vi "Get Actor Core Control Labels.vi"(8 "error in":errorcluster, 11 "Class in":refnum<class>) -> (0 "error out":errorcluster, 2 "Labels":string[](array[string]), 3 "Class out":refnum<class>)   [LabVIEW 2023, in "Label-Driven UI.lvlib"]
doc: "Actor Core.vi에 포함되어 있는 Nested in 컨트롤과 error in 컨트롤을 제외한 모든 컨트롤의 라벨들을 얻습니다."
uses:
  Label-Driven UI.lvlib
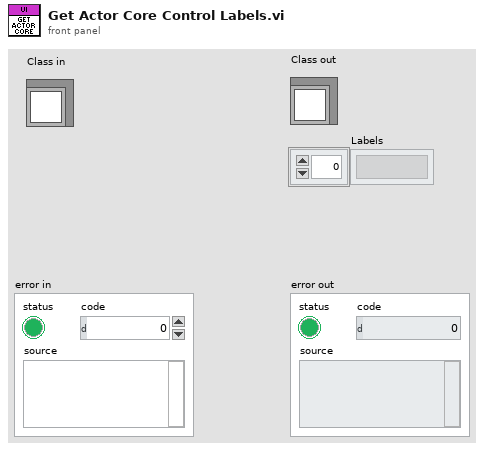
[diagram p1: front panel]
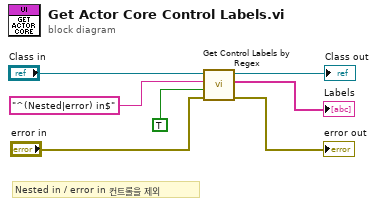
[diagram p0: block diagram]
diagram:
  # "Nested in / error in 컨트롤을 제외"
  n1 = call "Get Control Labels by Regex.vi"("error in"="error in", "Exclude? (F)"=TRUE ("Exclude?"), "regular expression"="^(Nested|error) in$", "Class in"="Class in") -> ("error out"=→"error out":errorcluster, "Labels"=→"Labels":string[], "Class out"=→"Class out":refnum<class>)  [unwired: 5 in]
